vi "StringSup.vi"(11 "String":string) -> (3 "result string":string)   [LabVIEW 2013]
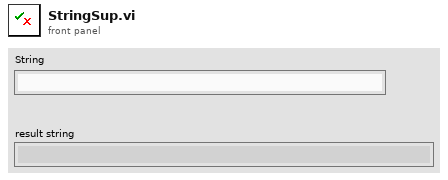
[diagram p1: front panel]
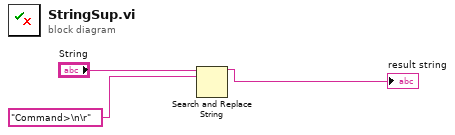
[diagram p0: block diagram]
diagram:
  n1 = Search and Replace String(input string="String", search string="Command>\n\r" ("substring (\"\")")) -> (result string=→"result string":string)  [unwired: 6 in, 3 out]
